vi "mtg - update graphs.vi"(8 "error in (no error)":errorcluster, 9 "new data":dbl[](array[numeric]), 10 "update list (10...)":i32[](array[numeric]), 11 "chart refs in":refnum<vi>[](array[refnum])) -> (0 "error out":errorcluster, 3 "chart refs out":refnum<vi>[](array[refnum]))   [LabVIEW 2025]
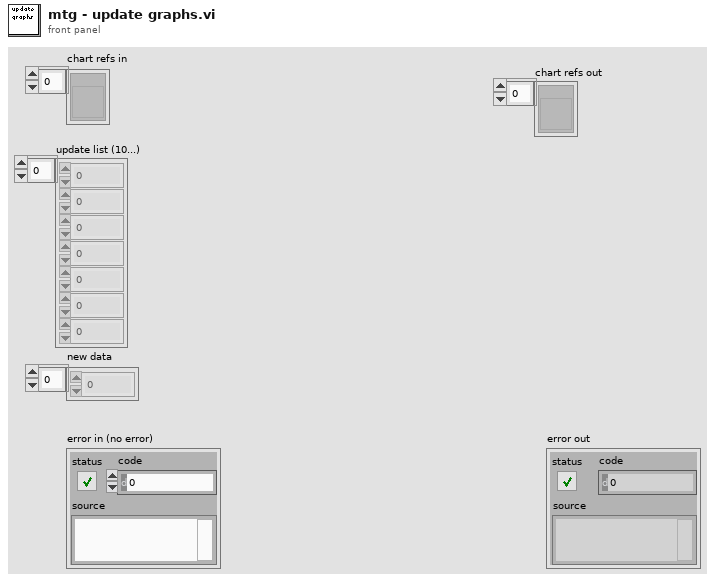
[diagram p1: front panel]
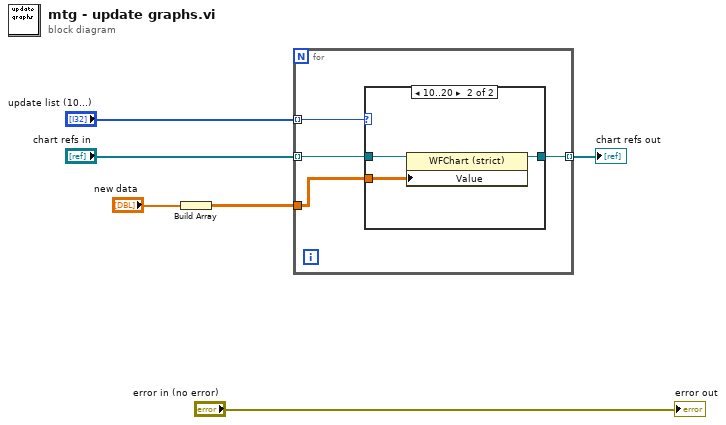
[diagram p0: block diagram]
diagram:
  n1 = Build Array("new data") -> (w1:dbl[][])
  n2 = for {
    tunnel: "chart refs in" -> [w10] mode=indexing
    tunnel: [w9] -> w4 mode=indexing
    tunnel: "update list (10...)" -> [w8] mode=indexing
    tunnel: w1 -> [w7]
    n3 = case shown="10..20" w8 {
      tunnel: w10 -> [w11 w14]
      tunnel: [w11 w13] -> w9
      tunnel: w7 -> [_ w12]
      frame 0, Default {
      }
      frame 10..20 {
        n4 = property class="WFChart (strict)"(reference=w14, "Value"=w12) -> (reference out=w13:refnum<vi>)  [unwired: 1 in, 1 out]
      }
    }
  }
  "chart refs out" <- w4
  "error out" <- "error in (no error)"
